vi "Configure Zoom Window.vi"(7 "Horizontal Position (50)":dbl=50.0, 8 "error in (no error)":errorcluster, 9 "Zoom Factor (0: X1)":i32(ring) items=["X1", "X2", "X5", "X10"], 10 "Enable Zoom (F: Disable)":bool, 11 "VISA resource name":refnum<visa-resource-name>) -> (0 "error out":errorcluster, 3 "VISA resource name out":refnum<visa-resource-name>)   [LabVIEW 2017, in "Tektronix TDS 200 1000 2000 Series.lvlib"]
doc: "Configures parameters related to zoom window.\n\n<B>Note(s):</b>\nAvailable on TBS1000B-EDU and TBS1000B series only."
uses:
  Tektronix TDS 200 1000 2000 Series.lvlib
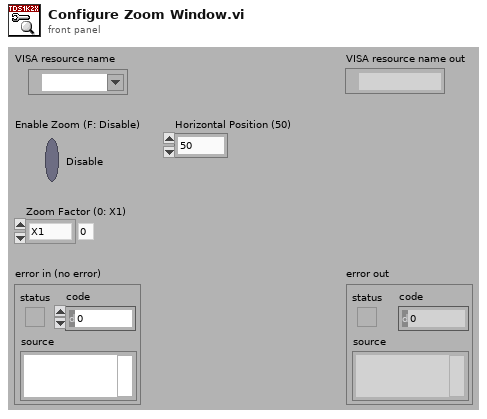
[diagram p1: front panel]
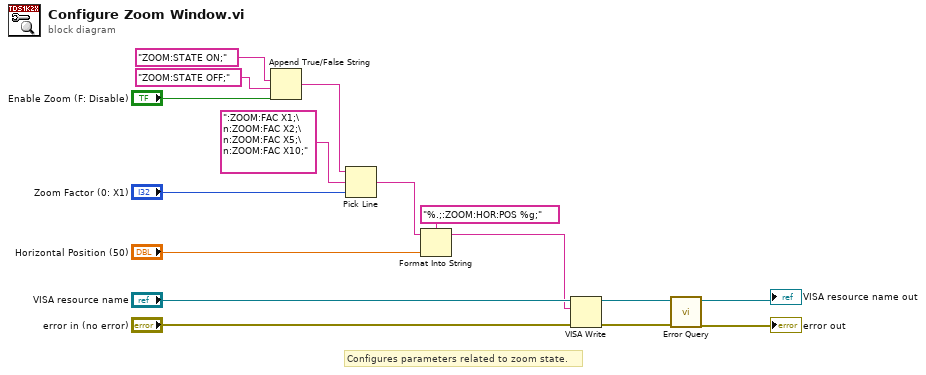
[diagram p0: block diagram]
diagram:
  # "Configures parameters related to zoom state."
  n1 = Append True/False String(1:"Enable Zoom (F: Disable)", 2:"ZOOM:STATE OFF;", 3:"ZOOM:STATE ON;") -> (0:w11:string)  [unwired: 1 out]
  n2 = Pick Line(string ("")=w11, multi-line string=":ZOOM:FAC X1;\n:ZOOM:FAC X2;\n:ZOOM:FAC X5;\n:ZOOM:FAC X10;", line index="Zoom Factor (0: X1)") -> (output string=w10:string)
  n3 = Format Into String(format string="%.;:ZOOM:HOR:POS %g;", initial string=w10, "Horizontal Position (50)") -> (resulting string=w1:string)  [unwired: 1 in, 1 out]
  n4 = VISA Write(VISA resource name="VISA resource name", write buffer=w1, error in (no error)="error in (no error)") -> (VISA resource name out=w6:refnum<visa-resource-name>, error out=w5:errorcluster)  [unwired: 1 out]
  n5 = call "Error Query.vi"("error in (no error)"=w5, "VISA resource name"=w6) -> ("error out"=→"error out":errorcluster, "VISA resource name out"=→"VISA resource name out":refnum<visa-resource-name>)  [unwired: 8 out]
